vi "Add to Array if Not Present (String).vi"(4 "String":string, 5 "String Array":string[](array[string])) -> (1 "New String Array":string[](array[string]))   [LabVIEW 2011]
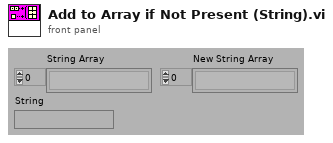
[diagram p1: front panel]
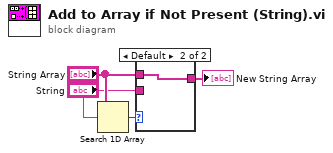
[diagram p0: block diagram]
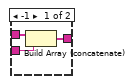
[diagram p2: hidden frame]
diagram:
  n1 = Search 1D Array(1D array="String Array", element="String") -> (index of element=w4:i32)  [unwired: 1 out]
  n2 = case shown="Default" w4 {
    tunnel: "String Array" -> [w7 w8]
    tunnel: "String" -> [w6 _]
    tunnel: [w5 w8] -> w1
    frame -1 {
      n3 = Build Array (concatenate)(w7, w6) -> (w5:string[])
    }
    frame Default {
    }
  }
  "New String Array" <- w1
